vi "GetMUXChannelNames.vi"(8 "error in (no error)":errorcluster, 10 "gRPCid":T2, 11 "ctet_mux in":T1) -> (0 "error out":errorcluster, 3 "ctet_mux out":T1)   [LabVIEW 2019, in "ctet_mux_User Library.lvlib"]
uses:
  ctet_mux_User Library.lvlib
  Servers/ctet_mux/gRPC lvSupport/Server API/typeDefs/grpcId.ctl
  Types/ctet_mux.ctl
  Servers/ctet_mux/ctet_mux Class/RPC Messages/measurementservice_ErrorOut/measurementservice_ErrorOut_Data.ctl
  Servers/ctet_mux/ctet_mux Class/RPC Messages/measurementservice_MUXGetChannelNamesResponse/measurementservice_MUXGetChannelNamesResponse_Data.ctl
  Servers/ctet_mux/ctet_mux Class/ctet_mux.lvclass
  Servers/ctet_mux/gRPC lvSupport/gprc-lvsupport.lvlib
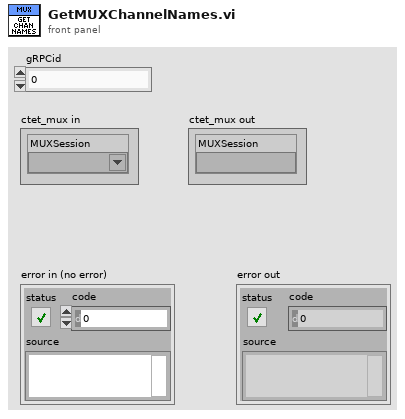
[diagram p1: front panel]
types:
  T1 = typedef "ctet_mux_User Library.lvlib/ctet_mux.ctl" = cluster{"MUXSession":refnum<k15>}
  T2 = typedef "ctet_mux.lvlib/gprc-lvsupport.lvlib/grpcId.ctl" = u64
  T3 = typedef "ctet_mux.lvlib/ctet_mux.lvclass/measurementservice_MUXGetChannelNamesResponse_Data.ctl" = cluster{"ChannelNames":string[], "error":T4}
  T4 = typedef "ctet_mux.lvlib/ctet_mux.lvclass/measurementservice_ErrorOut_Data.ctl" = cluster{"errCode":i64, "errMessage":string}
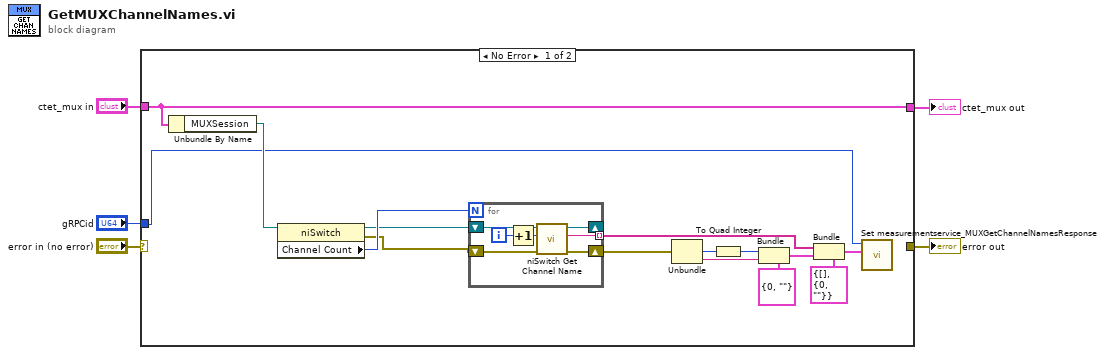
[diagram p0: block diagram]
diagram:
  n1 = case shown="No Error" "error in (no error)" {
    selector: "error in (no error)" -> [_ w29]
    tunnel: [_ w29] -> w5
    tunnel: "gRPCid" -> [w9 _]
    tunnel: "ctet_mux in" -> [w17 w28]
    tunnel: [w17 w28] -> w1
    frame No Error {
      n2 = Unbundle By Name(w17) -> ("MUXSession"=w15:refnum<k15>)
      n3 = property class="niSwitch"(reference=w15) -> (reference out=w13:refnum<k15>, error out=w12:errorcluster, "Channel Count"=w14:i32)  [unwired: 1 in]
      n4 = for {
        N: w14 -> [_]
        shift-right: [w24] -> _
        shift-left: w13 -> [w27]
        shift-right: [w25] -> w11
        shift-left: w12 -> [w26]
        tunnel: [w22] -> w6 mode=indexing
        i -> [w23]
        n5 = Increment(x=w23) -> (x+1=w21:i32)
        n6 = call <instrlib>:"niSwitch Get Channel Name.vi"("error in (no error)"=w26, "index (1)"=w21, "instrument handle"=w27) -> ("error out"=w25:errorcluster, "channel string"=w22:string, "instrument handle out"=w24:refnum<k15>)  [unwired: 6 in]
      }
      n7 = Unbundle(w11) -> ("code"=w19:i32, "source"=w20:string)  [unwired: 1 out]
      n8 = To Quad Integer(1:w19) -> (0:w18:i64)
      n9 = Bundle(cluster=T4 {"errCode"=0, "errMessage"=""} ("error"), "errCode"=w18, "errMessage"=w20) -> (w7:T4)
      n10 = Bundle(cluster=T3 {"ChannelNames"=[], "error"={"errCode"=0, "errMessage"=""}} ("measurementservice_MUXGetChannelNamesResponse_Data"), "ChannelNames"=w6, "error"=w7) -> (w8:T3)
      n11 = call "Set measurementservice_MUXGetChannelNamesResponse.vi"("Message Data"=w8, "gRPCid"=w9) -> ()  [unwired: 9 in, 1 out]
    }
    frame Error {
    }
  }
  "error out" <- w5
  "ctet_mux out" <- w1
